vi "WPI_DashboardUpdateCameraIndices.vi"(10 "Display Index":u32, 11 "Numeric":i32) -> ()   [LabVIEW 2025]
uses:
  <vilib>/Rock Robotics/WPI/Dashboard/WPI_DashboardLogging Global.vi
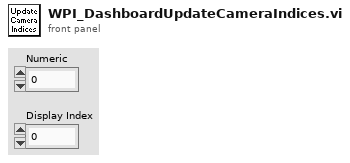
[diagram p1: front panel]
types:
  T1 = cluster{"Video 1":i32, "Video 2":i32, "Video 3":i32, "Video 4":i32}
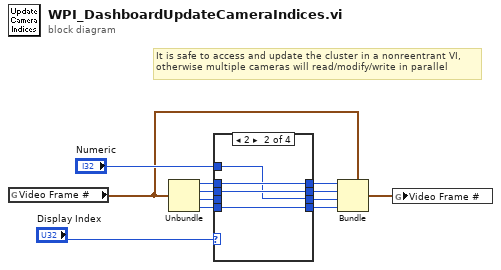
[diagram p0: block diagram]
diagram:
  # "It is safe to access and update the cluster in a nonreentrant VI,\notherwise multiple cameras will read/modify/write in parallel"
  n1 = global read "WPI_DashboardLogging Global.vi" "Video Frame #"() -> (w6:T1)
  n2 = Unbundle(w6) -> ("Video 1"=w11:i32, "Video 2"=w10:i32, "Video 3"=w9:i32, "Video 4"=w8:i32)
  n3 = case shown="2" "Display Index" {
    tunnel: w11 -> [_ w20 w24 w28]
    tunnel: w10 -> [w16 w19 w23 _]
    tunnel: w9 -> [w15 _ w22 w27]
    tunnel: w8 -> [w14 w18 _ w26]
    tunnel: "Numeric" -> [w13 w17 w21 w25]
    tunnel: [w13 w20 w24 w28] -> w5
    tunnel: [w16 w19 w23 w25] -> w3
    tunnel: [w15 w17 w22 w27] -> w2
    tunnel: [w14 w18 w21 w26] -> w1
    frame 0, Default {
    }
    frame 2 {
    }
    frame 3 {
    }
    frame 1 {
    }
  }
  n4 = Bundle(cluster=w6, "Video 1"=w5, "Video 2"=w3, "Video 3"=w2, "Video 4"=w1) -> (w4:T1)
  n5 = global write "WPI_DashboardLogging Global.vi" "Video Frame #"(w4) -> ()
